vi "Fit.vi"(8 "error in (no error)":errorcluster caption="entrée d'erreur (pas d'erreur)", 9 "y":string[][](array[string]), 10 "X":string[][](array[string]), 11 "KNNImputer.lvclass":refnum<class "KNNImputer.lvclass">) -> (0 "error out":errorcluster caption="sortie d'erreur", 2 "String Data":string, 3 "KNNImputer.lvclass":refnum<class "KNNImputer.lvclass">)   [LabVIEW 2020, in "KNNImputer.lvclass"]
doc: "Fit the imputer on X.\n\nReturns : \n\n- String : OK"
uses:
  KNNImputer.lvclass
  KNNImputer.lvclass/KNNImputer.ctl
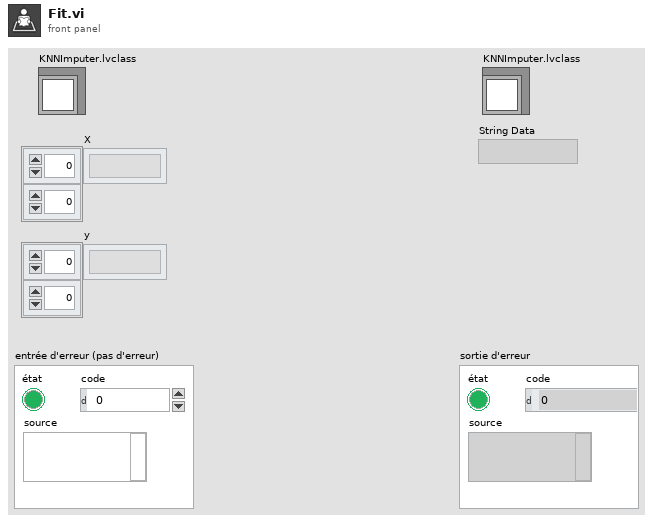
[diagram p1: front panel]
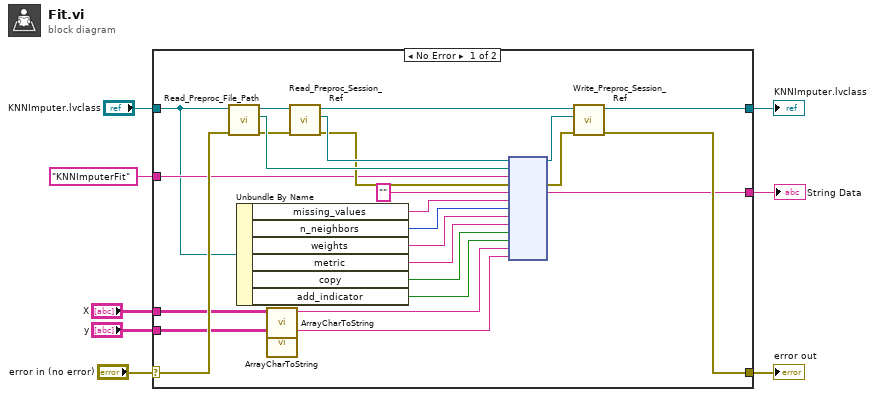
[diagram p0: block diagram]
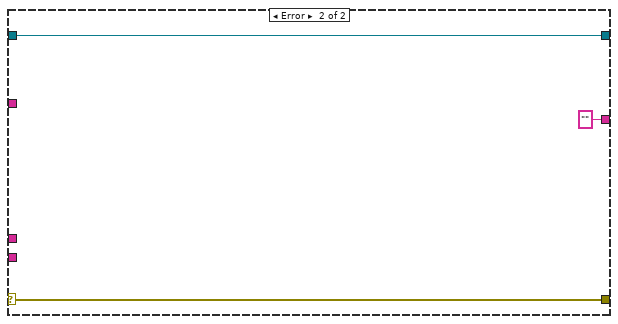
[diagram p2: hidden frame]
diagram:
  n1 = case shown="No Error" "error in (no error)" {
    selector: "error in (no error)" -> [w24 w36]
    tunnel: [w23 w36] -> w7
    tunnel: [w22 w35] -> w5
    tunnel: "KNNImputer.lvclass" -> [w19 w35]
    tunnel: "KNNImputerFit" ("Fonction") -> [w21 _]
    tunnel: [w20 ""] -> w3
    tunnel: "X" -> [w12 _]
    tunnel: "y" -> [w10 _]
    frame No Error {
      n2 = call-dynamic "Read_Preproc_File_Path.vi"("error in (no error)"=w24, "Python in"=w19) -> ("error out"=w28:errorcluster, "File_Path"=w31:path, "Python out"=w33:refnum<class "KNNImputer.lvclass">)  [unwired: 7 in]
      n3 = Unbundle By Name(w19) -> ("missing_values"=w18:string, "n_neighbors"=w17:i32, "weights"=w16:string, "metric"=w15:string, "copy"=w14:bool, "add_indicator"=w13:bool)
      n4 = call "ArrayCharToString.vi"("TAB"=w12) -> ("Instruction"=w11:string)  [unwired: 10 in]
      n5 = call "ArrayCharToString.vi"("TAB"=w10) -> ("Instruction"=w9:string)  [unwired: 10 in]
      n6 = call-dynamic "Read_Preproc_Session_Ref.vi"("error in (no error)"=w28, "Python in"=w33) -> ("error out"=w29:errorcluster, "Session_ref"=w30:refnum<k35>, "Python out"=w32:refnum<class "KNNImputer.lvclass">)  [unwired: 7 in]
      n7 = node(w30, w31, w21, w29, "", w18, w17, w16, w15, w14, w13, w11, w9) -> (w25:refnum<k35>, w27:errorcluster, w20:string)  [unwired: 8 in, 2 out]
      n8 = call-dynamic "Write_Preproc_Session_Ref.vi"("error in (no error)"=w27, "Session_ref"=w25, "Python in"=w32) -> ("error out"=w23:errorcluster, "Python out"=w22:refnum<class "KNNImputer.lvclass">)  [unwired: 7 in]
    }
    frame Error {
    }
  }
  "error out" <- w7
  "KNNImputer.lvclass" <- w5
  "String Data" <- w3
